vi "WriteToCSVFromNT.vi"() -> ()   [LabVIEW 2019]
uses:
  <vilib>/Rock Robotics/Network Tables/NT Read String Array.vi
  <vilib>/Utility/file.llb/Write Delimited Spreadsheet (string).vi
  CalibrationsGlobalVariables.vi
panel:
  in  "Enum 3":T1(ring)
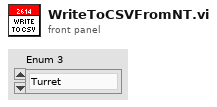
[diagram p1: front panel]
types:
  T1 = enum16{"Turret", "Magazine", "Intake", "Flywheel", "Drive", "Control_Panel_"}
  T2 = enum16{"open", "replace", "create", "open or create", "replace or create", "replace or create with confirmation"}
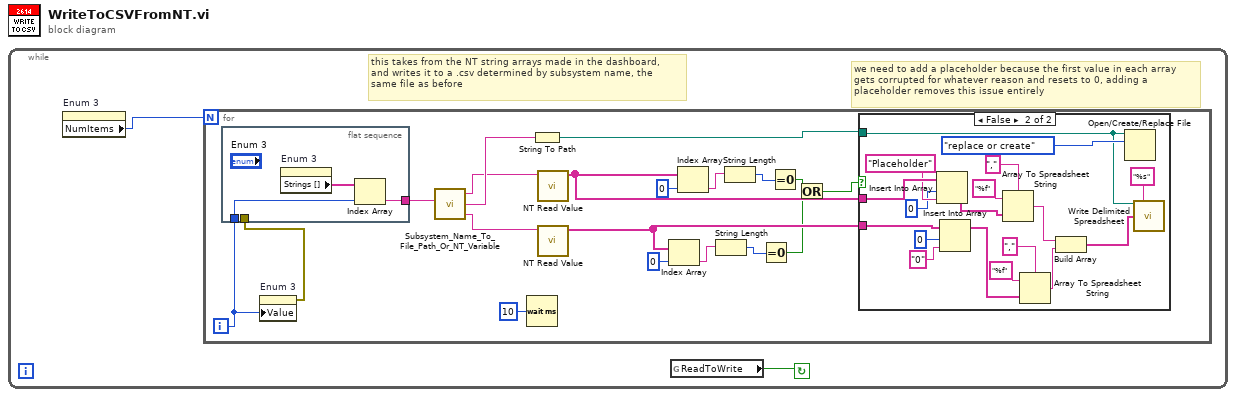
[diagram p0: block diagram]
diagram:
  n1 = while {
    stop <- w1 continue-if-true
    # "we need to add a placeholder because the first value in each array\ngets corrupted for whatever reason and resets to 0, adding a\nplaceholder removes this issue entirely"
    # "this takes from the NT string arrays made in the dashboard, \nand writes it to a .csv determined by subsystem name, the\nsame file as before"
    n2 = property on="Enum 3" class="Enum (strict)"() -> ("NumItems"=w2:u32)  [unwired: 2 in, 2 out]
    n3 = for {
      N: w2 -> [_]
      i -> [w20]
      n4 = flat-sequence {
        tunnel: w21 -> [_]
        tunnel: w20 -> [w41]
        tunnel: [w40] -> w16
        frame #0 {
          n5 = property on="Enum 3" class="Enum (strict)"() -> ("Strings []"=w42:string[])  [unwired: 2 in, 2 out]
          n6 = Index Array(array=w42, index=w41) -> (element=w40:string)
        }
      }
      n7 = property on="Enum 3" class="Enum (strict)"("Value"=w20) -> (error out=w21:errorcluster)  [unwired: 2 in, 1 out]
      n8 = call "Subsystem_Name_To_File_Path_Or_NT_Variable.vi"("Enum String Name"=w16) -> ("Names"=w14:string, "File Path"=w18:string, "Values"=w19:string)  [unwired: 5 in]
      n9 = Wait (ms)(milliseconds to wait=u32 10) -> ()  [unwired: 1 out]
      n10 = String To Path(string=w18) -> (path=w17:path)
      n11 = call-poly <vilib>:"NT Read Value.vi"("Name"=w14) -> ("String Array"=w13:string[])  [unwired: 9 in, 1 out]
      n12 = call-poly <vilib>:"NT Read Value.vi"("Name"=w19) -> ("String Array"=w6:string[])  [unwired: 9 in, 1 out]
      n13 = Index Array(array=w6, index=0) -> (element=w8:string)
      n14 = Index Array(array=w13, index=0) -> (element=w11:string)
      n15 = String Length(string=w8) -> (length=w7:i32)
      n16 = String Length(string=w11) -> (length=w10:i32)
      n17 = Equal To 0?(x=w7) -> (x = 0?=w4:bool)
      n18 = Equal To 0?(x=w10) -> (x = 0?=w5:bool)
      n19 = Or(x=w5, y=w4) -> (x .or. y?=w3:bool)
      n20 = case shown="False" w3 {
        tunnel: w17 -> [_ w33]
        tunnel: w13 -> [_ w28]
        tunnel: w6 -> [_ w29]
        frame True {
        }
        frame False {
          n21 = Insert Into Array(array=w28, index=0, new element="Placeholder" ("new element/subarray")) -> (w25:string[])
          n22 = Insert Into Array(array=w29, index=0, new element="0" ("new element/subarray")) -> (w24:string[])
          n23 = Array To Spreadsheet String(delimiter (Tab)=",", array=w25, 3:"%f" ("format string")) -> (spreadsheet string=w35:string)
          n24 = Array To Spreadsheet String(delimiter (Tab)=",", array=w24, 3:"%f" ("format string")) -> (spreadsheet string=w32:string)
          n25 = Build Array(w35, w32) -> (w31:string[])
          n26 = Open/Create/Replace File(file path (use dialog)=w33, operation (0:open)=T2."replace or create") -> ()  [unwired: 4 in, 3 out]
          n27 = call-poly <vilib>:"Write Delimited Spreadsheet.vi"("file path (dialog if empty)"=w33, "format (%s)"="%s", "1D data"=w31) -> ()  [unwired: 11 in, 2 out]
        }
      }
    }
    n28 = global read "CalibrationsGlobalVariables.vi" "ReadToWrite"() -> (w1:bool)
  }
